vi "Display Unicode Tab Control Page Tabs.vi"() -> ()   [LabVIEW 2009]
panel:
  in  "Language":u16(ring) items=["English", "Japanese", "Chinese"]
  in  "Tab Control":enum32{"Page 1", "Page 2", "Page 3"}(tab) caption="h~{§c6R"
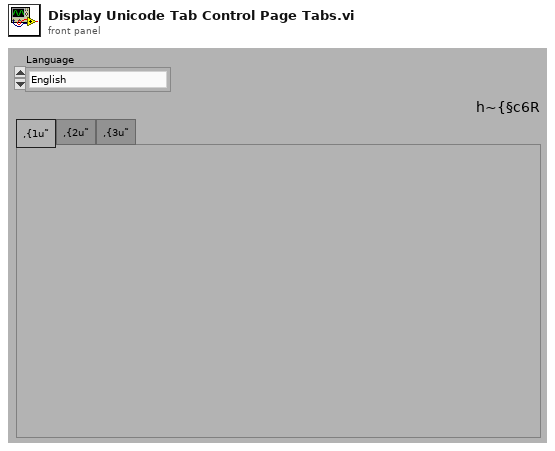
[diagram p1: front panel]
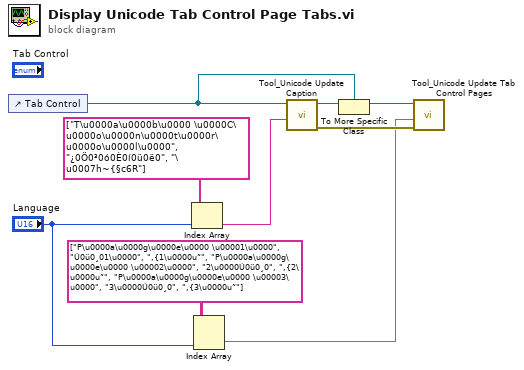
[diagram p0: block diagram]
diagram:
  n1 = control-ref of="Tab Control"() -> (w2:refnum<vi>)
  n2 = Index Array(array=string[] ["T\u0000a\u0000b\u0000 \u0000C\u0000o\u0000n\u0000t\u0000r\u0000o\u0000l\u0000", "¿0Ö0³0ó0È0í0ü0ë0", "\u0007h~{§c6R"], index="Language") -> (element=w8:string)
  n3 = Index Array(array=string[][] [["P\u0000a\u0000g\u0000e\u0000 \u00001\u0000", "Ú0ü0¸01\u0000", ",{1\u0000u˜"], ["P\u0000a\u0000g\u0000e\u0000 \u00002\u0000", "2\u0000Ú0ü0¸0", ",{2\u0000u˜"], ["P\u0000a\u0000g\u0000e\u0000 \u00003\u0000", "3\u0000Ú0ü0¸0", ",{3\u0000u˜"]], index (col)="Language") -> (element=w1:string[])  [unwired: 1 in]
  n4 = call "Tool_Unicode Update Caption.vi"("Caption"=w8, "Control Reference"=w2) -> ("error out"=w6:errorcluster, "Control Reference"=w4:refnum<vi>)  [unwired: 6 in]
  n5 = To More Specific Class(target class=w2, reference=w4) -> (specific class reference=w3:refnum<vi>)  [unwired: 1 in, 1 out]
  n6 = call "Tool_Unicode Update Tab Control Pages.vi"("error in"=w6, "Page Captions"=w1, "Tab Control"=w3) -> ()  [unwired: 5 in, 2 out]
